vi "Coral Immediate.vi"(4 "Positional Array":dbl[](array[numeric]), 6 "Setpoint State":T1=enum."L2", 7 "Description":string, 8 "Command Info In":T4, 9 "Confirm or Negate":bool, 10 "Coral States":T2, 11 "Operation":T3) -> (0 "Command Info Out":T4)   [LabVIEW 2023]
doc: "This template is useful for immediate subsystem actions that do not need deadband filtering\n\nBe sure to right-click and select New from Template and save with a new command name."
uses:
  <vilib>/Rock Robotics/WPI/Framework/Command Status Info.ctl
  <vilib>/Rock Robotics/WPI/Framework/Completion Status.ctl
  <vilib>/Rock Robotics/WPI/Framework/Completion Notifier.ctl
  Implementation/Coral Operations.ctl
  Support Code/Teleop Util/Coral States.ctl
  Support Code/Teleop Util/Scoring Levels.ctl
  Implementation/Coral Setpoints.ctl
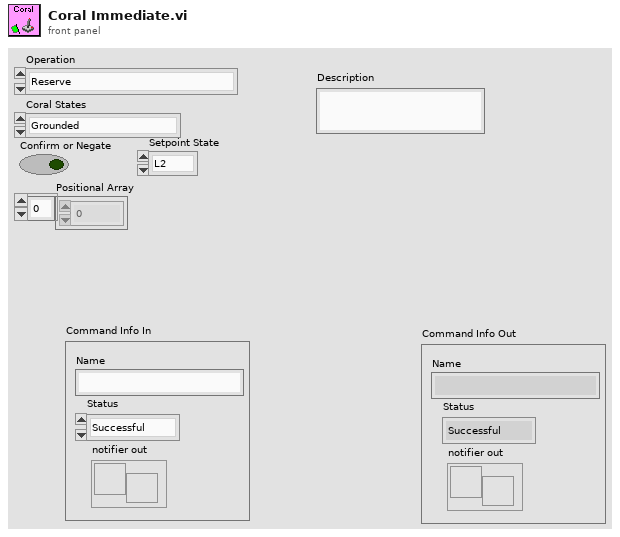
[diagram p1: front panel]
types:
  T1 = typedef "Scoring Levels.ctl" = enum16{"Trough", "L2", "L3", "L4", "Default"}
  T2 = typedef "Coral States.ctl" = enum16{"Grounded", "Coral Intake", "Scoring Sequence", "Hold Position", "Score", "Manual Override", "Climb Safety Mode"}
  T3 = typedef "Coral Operations.ctl" = enum16{"Reserve", "Read Current", "Immediate", "Calibrate"}
  T4 = typedef "Command Status Info.ctl" = cluster{"Name":string, "Status":T5, "notifier out":T6}
  T5 = typedef "Completion Status.ctl" = enum16{"Successful", "Aborted", "Incomplete"}
  T6 = typedef "Completion Notifier.ctl" = refnum<notifier>
  T7 = typedef "Coral Setpoints.ctl" = cluster{"Operation":T3, "Coral States":T2, "Confirm or Negate":bool, "Positional Array":dbl[], "Setpoint State":T1}
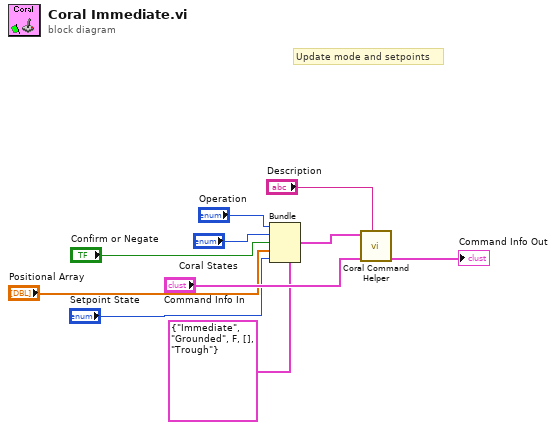
[diagram p0: block diagram]
diagram:
  # "Update mode and setpoints"
  n1 = Bundle(cluster=T7 {"Operation"=enum."Immediate", "Coral States"=enum."Grounded", "Confirm or Negate"=FALSE, "Positional Array"=[], "Setpoint State"=enum."Trough"} ("SubSystem Data"), "Operation"="Operation", "Coral States"="Coral States", "Confirm or Negate"="Confirm or Negate", "Positional Array"="Positional Array", "Setpoint State"="Setpoint State") -> (w6:T7)
  n2 = call "Coral Command Helper.vi"("Description"="Description", "Command Info In"="Command Info In", "SubSystem Data"=w6) -> ("Command Info Out"=→"Command Info Out":T4)  [unwired: 6 in, 2 out]
